vi "PLC Off.vi"(8 "error in (no error)":errorcluster, 11 "Programming Logicv2 in":refnum<class "Programming Logicv2.lvclass">) -> (0 "error out":errorcluster, 3 "Programming Logicv2 out":refnum<class "Programming Logicv2.lvclass">)   [LabVIEW 2014, in "Main Libraryv2.lvlib" / "Programming Logicv2.lvclass"]
uses:
  Programming Logicv2.lvclass
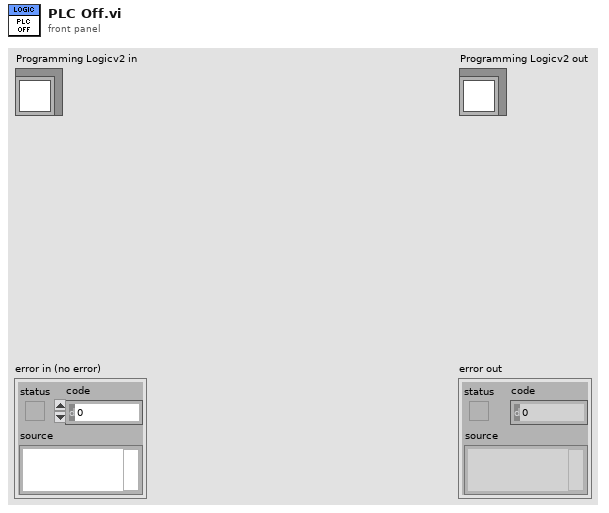
[diagram p1: front panel]
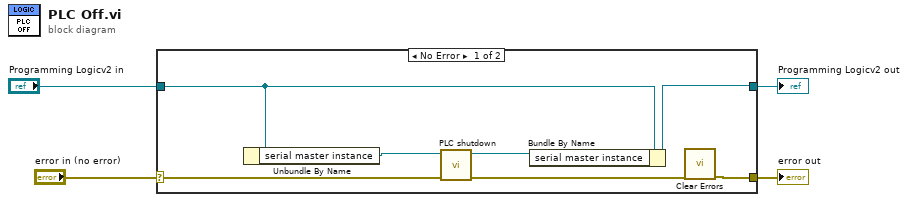
[diagram p0: block diagram]
diagram:
  n1 = case shown="No Error" "error in (no error)" {
    selector: "error in (no error)" -> [w11 w13]
    tunnel: [w6 w13] -> w3
    tunnel: [w8 w12] -> w1
    tunnel: "Programming Logicv2 in" -> [w9 w12]
    frame No Error {
      n2 = Unbundle By Name(w9) -> ("serial master instance"=w10:refnum<class "Modbus Master.lvclass">)
      n3 = call "PLC shutdown.vi"("error in"=w11, "Modbus master in"=w10) -> ("error out"=w5:errorcluster, "Modbus master out"=w7:refnum<class "Modbus Master.lvclass">)  [unwired: 8 in]
      n4 = Bundle By Name(cluster=w9, "serial master instance"=w7) -> (w8:refnum<class "Programming Logicv2.lvclass">)
      n5 = call <vilib>:"Clear Errors.vi"("error in (no error)"=w5) -> ("error out"=w6:errorcluster)  [unwired: 5 in, 1 out]
    }
    frame Error {
    }
  }
  "error out" <- w3
  "Programming Logicv2 out" <- w1
